vi "TargetCorner_Equals.vi"(9 "Other TargetCorner":T1, 11 "TargetCorner":T1) -> (3 "Equals":bool)   [LabVIEW 2019, in "PhotonVisionLib.lvlib"]
doc: "Determines if two target corners are equal\n\nInputs:\n - TargetCorner -- TargetCorner cluster\n - OtherTargetCorner -- TargetConrer cluster to compare\n\nOutputs:\n - Equals -- TRUE if both TargetCorners are equal"
uses:
  PhotonVisionLib.lvlib
  TypeDef/TargetCornerType.ctl
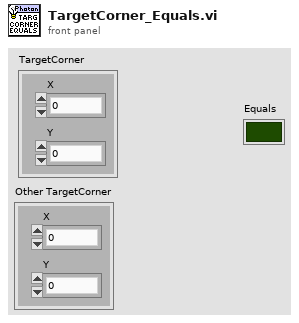
[diagram p1: front panel]
types:
  T1 = typedef "PhotonVisionLib.lvlib/TargetCornerType.ctl" = cluster{"X":dbl, "Y":dbl}
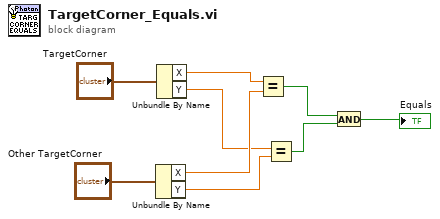
[diagram p0: block diagram]
diagram:
  n1 = Unbundle By Name("Other TargetCorner") -> ("X"=w6:dbl, "Y"=w4:dbl)
  n2 = Unbundle By Name("TargetCorner") -> ("X"=w7:dbl, "Y"=w5:dbl)
  n3 = Equal?(x=w7, y=w6) -> (x = y?=w2:bool)
  n4 = Equal?(x=w5, y=w4) -> (x = y?=w3:bool)
  n5 = And(x=w2, y=w3) -> (x .and. y?=→"Equals":bool)
